vi "SaveResults.vi"(8 "Error In":errorcluster, 9 "Result 2":u64, 10 "Result 2":u64) -> (0 "Error Out":errorcluster)   [LabVIEW 2020, in "AdventCode.lvclass"]
uses:
  AdventCode.lvclass
  AdventCode.lvclass/AdventCode.ctl
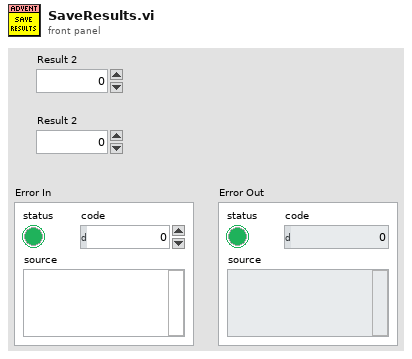
[diagram p1: front panel]
types:
  T1 = typedef "AdventCode.lvclass/ObjectAttributes.ctl" = cluster{"Year":i32, "Day":i32, "PuzzleData":string}
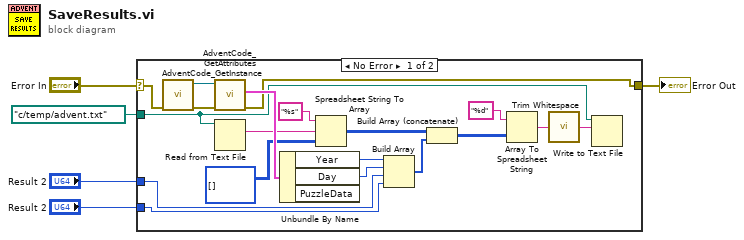
[diagram p0: block diagram]
diagram:
  n1 = case shown="No Error" "Error In" {
    selector: "Error In" -> [w21 w25]
    tunnel: [w23 w25] -> w4
    tunnel: path "c:/temp/advent.txt" -> [w9 _]
    tunnel: "Result 2" -> [w13 _]
    tunnel: "Result 2" -> [w6 _]
    frame No Error {
      n2 = call "AdventCode_GetInstance.vi"("error in"=w21) -> ("error out"=w20:errorcluster, "reference out"=w22:refnum<class "AdventCode.lvclass">)  [unwired: 6 in, 3 out]
      n3 = call "AdventCode_GetAttributes.vi"("error in (no error)"=w20, "reference in"=w22) -> ("error out"=w23:errorcluster, "Data"=w24:T1)  [unwired: 6 in, 2 out]
      n4 = Read from Text File(file (use dialog)=w9) -> (text=w19:string)  [unwired: 3 in, 3 out]
      n5 = Unbundle By Name(w24) -> ("Year"=w15:i32, "Day"=w14:i32)  [unwired: 1 out]
      n6 = Spreadsheet String To Array(format string="%s", spreadsheet string=w19, array type (2D Dbl)=i32[][] []) -> (array=w16:i32[][])  [unwired: 1 in]
      n7 = Build Array(w15, w14, w13, w6) -> (w12:u64[])
      n8 = Build Array (concatenate)(w16, w12) -> (w11:u64[][])
      n9 = Array To Spreadsheet String(array=w11, 3:"%d" ("format string")) -> (spreadsheet string=w8:string)  [unwired: 1 in]
      n10 = call <vilib>:"Trim Whitespace.vi"("string"=w8) -> ("trimmed string"=w7:string)  [unwired: 1 in]
      n11 = Write to Text File(file (use dialog)=w9, text=w7) -> ()  [unwired: 2 in, 3 out]
    }
    frame Error {
    }
  }
  "Error Out" <- w4
